vi "根据下拉框显示参数.vi"(0 "refnum":T1, 1 "Ring引用句柄":refnum<vi>, 2 "参数引用句柄":refnum<vi>, 3 "error in (no error)":errorcluster) -> (7 "引用句柄输出":T1 caption="refnum out", 10 "error out":errorcluster caption="错误输出")   [LabVIEW 2015]
uses:
  <vilib>/Utility/config.llb/Config Data RefNum.ctl
  <vilib>/Utility/config.llb/Read Key (String).vi
  <vilib>/Utility/config.llb/Read Key (U32).vi
  <vilib>/Utility/config.llb/NI_LVConfig.lvlib
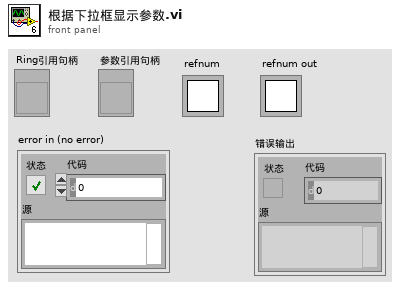
[diagram p1: front panel]
types:
  T1 = typedef "NI_LVConfig.lvlib/Config Data RefNum.ctl" = refnum<k1>
  T2 = typedef "GPRS参数123.ctl" = cluster{"IP地址":string, "端口号":u16, "工作模式":u16, "连接协议":u16, "连接方式":u16, "本机号码":string, "短信监控中心号码1":string, "监听时间":u16, "心跳间隔":u16, "重启时间(分)":u16, "C/S关系":u16, "DNS域名":string, "APN接入点":string, "报头使能":u16, "ID号":string, "波特率":u16, "数据位":u16, "停止位":u16, "校验位":u16, "短信目标号码1 ":string, "短信目标号码2":string, "短信监控中心号码2":string, "信号检测使能":u16, "控制方式":u16}
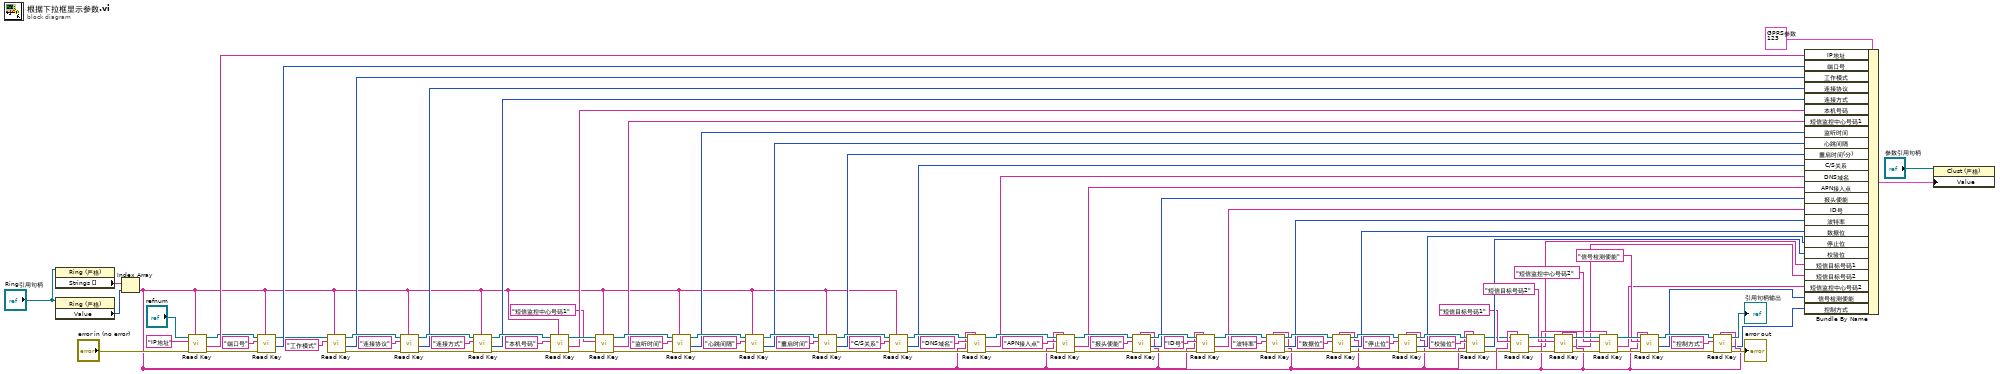
[diagram p0: block diagram]
diagram:
  n1 = property class="Ring (严格)"(reference="Ring引用句柄") -> ("Strings []"=w102:string[])  [unwired: 1 in, 2 out]
  n2 = property class="Ring (严格)"(reference="Ring引用句柄") -> ("Value"=w101:u16)  [unwired: 1 in, 2 out]
  n3 = Index Array(array=w102, index=w101) -> (element=w9:string)
  n4 = call-poly <vilib>:"Read Key.vi"("section"=w9, "error in (no error)"="error in (no error)", "key"="IP地址", "refnum"="refnum") -> ("error out"=w94:errorcluster, "value"=w96:string, "refnum out"=w95:T1)  [unwired: 4 in, 1 out]
  n5 = call-poly <vilib>:"Read Key.vi"("section"=w9, "error in (no error)"=w94, "key"="端口号", "refnum"=w95) -> ("value"=w92:u32, "refnum out"=w71:T1)  [unwired: 4 in, 2 out]
  n6 = call-poly <vilib>:"Read Key.vi"("section"=w9, "key"="工作模式", "refnum"=w71) -> ("error out"=w91:errorcluster, "value"=w73:u32, "refnum out"=w90:T1)  [unwired: 5 in, 1 out]
  n7 = call-poly <vilib>:"Read Key.vi"("section"=w9, "error in (no error)"=w91, "key"="连接协议", "refnum"=w90) -> ("error out"=w75:errorcluster, "value"=w72:u32, "refnum out"=w74:T1)  [unwired: 4 in, 1 out]
  n8 = call-poly <vilib>:"Read Key.vi"("section"=w9, "error in (no error)"=w75, "key"="连接方式", "refnum"=w74) -> ("error out"=w89:errorcluster, "value"=w56:u32, "refnum out"=w88:T1)  [unwired: 4 in, 1 out]
  n9 = call-poly <vilib>:"Read Key.vi"("section"=w9, "error in (no error)"=w89, "key"="本机号码", "refnum"=w88) -> ("error out"=w69:errorcluster, "value"=w55:string, "refnum out"=w70:T1)  [unwired: 4 in, 1 out]
  n10 = call-poly <vilib>:"Read Key.vi"("section"=w9, "error in (no error)"=w69, "key"="短信监控中心号码1", "refnum"=w70) -> ("error out"=w87:errorcluster, "value"=w54:string, "refnum out"=w86:T1)  [unwired: 4 in, 1 out]
  n11 = call-poly <vilib>:"Read Key.vi"("section"=w9, "error in (no error)"=w87, "key"="监听时间", "refnum"=w86) -> ("error out"=w67:errorcluster, "value"=w48:u32, "refnum out"=w68:T1)  [unwired: 4 in, 1 out]
  n12 = call-poly <vilib>:"Read Key.vi"("section"=w9, "error in (no error)"=w67, "key"="心跳间隔", "refnum"=w68) -> ("error out"=w85:errorcluster, "value"=w47:u32, "refnum out"=w84:T1)  [unwired: 4 in, 1 out]
  n13 = call-poly <vilib>:"Read Key.vi"("section"=w9, "error in (no error)"=w85, "key"="重启时间", "refnum"=w84) -> ("error out"=w66:errorcluster, "value"=w46:u32, "refnum out"=w65:T1)  [unwired: 4 in, 1 out]
  n14 = call-poly <vilib>:"Read Key.vi"("section"=w9, "error in (no error)"=w66, "key"="C/S关系", "refnum"=w65) -> ("error out"=w83:errorcluster, "value"=w45:u32, "refnum out"=w82:T1)  [unwired: 4 in, 1 out]
  n15 = call-poly <vilib>:"Read Key.vi"("section"=w9, "error in (no error)"=w83, "key"="DNS域名", "refnum"=w82) -> ("error out"=w64:errorcluster, "value"=w44:string, "refnum out"=w63:T1)  [unwired: 4 in, 1 out]
  n16 = call-poly <vilib>:"Read Key.vi"("section"=w9, "error in (no error)"=w64, "key"="APN接入点", "refnum"=w63) -> ("error out"=w81:errorcluster, "value"=w43:string, "refnum out"=w80:T1)  [unwired: 4 in, 1 out]
  n17 = call-poly <vilib>:"Read Key.vi"("section"=w9, "error in (no error)"=w81, "key"="报头使能", "refnum"=w80) -> ("error out"=w62:errorcluster, "value"=w36:u32, "refnum out"=w61:T1)  [unwired: 4 in, 1 out]
  n18 = call-poly <vilib>:"Read Key.vi"("section"=w9, "error in (no error)"=w62, "key"="ID号", "refnum"=w61) -> ("error out"=w79:errorcluster, "value"=w35:string, "refnum out"=w78:T1)  [unwired: 4 in, 1 out]
  n19 = call-poly <vilib>:"Read Key.vi"("section"=w9, "error in (no error)"=w79, "key"="波特率", "refnum"=w78) -> ("error out"=w60:errorcluster, "value"=w32:u32, "refnum out"=w59:T1)  [unwired: 4 in, 1 out]
  n20 = call-poly <vilib>:"Read Key.vi"("section"=w9, "error in (no error)"=w60, "key"="数据位", "refnum"=w59) -> ("error out"=w77:errorcluster, "value"=w31:u32, "refnum out"=w76:T1)  [unwired: 4 in, 1 out]
  n21 = call-poly <vilib>:"Read Key.vi"("section"=w9, "error in (no error)"=w77, "key"="停止位", "refnum"=w76) -> ("error out"=w57:errorcluster, "value"=w28:u32, "refnum out"=w58:T1)  [unwired: 4 in, 1 out]
  n22 = call-poly <vilib>:"Read Key.vi"("section"=w9, "error in (no error)"=w57, "key"="校验位", "refnum"=w58) -> ("error out"=w8:errorcluster, "value"=w27:u32, "refnum out"=w7:T1)  [unwired: 4 in, 1 out]
  n23 = call-poly <vilib>:"Read Key.vi"("section"=w9, "error in (no error)"=w8, "key"="短信目标号码1", "refnum"=w7) -> ("error out"=w22:errorcluster, "value"=w1:string, "refnum out"=w23:T1)  [unwired: 4 in, 1 out]
  n24 = call-poly <vilib>:"Read Key.vi"("section"=w9, "error in (no error)"=w22, "key"="短信目标号码2", "refnum"=w23) -> ("error out"=w25:errorcluster, "value"=w2:string, "refnum out"=w24:T1)  [unwired: 4 in, 1 out]
  n25 = call-poly <vilib>:"Read Key.vi"("section"=w9, "error in (no error)"=w25, "key"="短信监控中心号码2", "refnum"=w24) -> ("error out"=w19:errorcluster, "value"=w3:string, "refnum out"=w18:T1)  [unwired: 4 in, 1 out]
  n26 = call-poly <vilib>:"Read Key.vi"("section"=w9, "error in (no error)"=w19, "key"="信号检测使能", "refnum"=w18) -> ("error out"=w13:errorcluster, "value"=w6:u32, "refnum out"=w14:T1)  [unwired: 4 in, 1 out]
  n27 = call-poly <vilib>:"Read Key.vi"("section"=w9, "error in (no error)"=w13, "key"="控制方式", "refnum"=w14) -> ("error out"=→"error out":errorcluster, "value"=w5:u32, "refnum out"=→"引用句柄输出":T1)  [unwired: 4 in, 1 out]
  n28 = Bundle By Name(cluster=T2 {"IP地址"="192.168.1.1", "端口号"=5070, "工作模式"=48, "连接协议"=48, "连接方式"=48, "本机号码"="13806871122", "短信监控中心号码1"="13800577500", "监听时间"=0, "心跳间隔"=0, "重启时间(分)"=0, "C/S关系"=48, "DNS域名"="", "APN接入点"="", "报头使能"=48, "ID号"="\u00124Vx", "波特率"=45060, "数据位"=56, "停止位"=49, "校验位"=48, "短信目标号码1 "="", "短信目标号码2"="", "短信监控中心号码2"="", "信号检测使能"=48, "控制方式"=48} ("GPRS参数（科技）"), "IP地址"=w96, "端口号"=w92, "工作模式"=w73, "连接协议"=w72, "连接方式"=w56, "本机号码"=w55, "短信监控中心号码1"=w54, "监听时间"=w48, "心跳间隔"=w47, "重启时间(分)"=w46, "C/S关系"=w45, "DNS域名"=w44, "APN接入点"=w43, "报头使能"=w36, "ID号"=w35, "波特率"=w32, "数据位"=w31, "停止位"=w28, "校验位"=w27, "短信目标号码1"=w1, "短信目标号码2"=w2, "短信监控中心号码2"=w3, "信号检测使能"=w6, "控制方式"=w5) -> (w97:T2)
  n29 = property class="Clust (严格)"(reference="参数引用句柄", "Value"=w97) -> ()  [unwired: 1 in, 2 out]
